vi "Self-Test.vi"(8 "error in (no error)":errorcluster, 11 "VISA resource name":refnum<visa-resource-name>) -> (0 "error out":errorcluster, 1 "Self-Test Result Message":string, 2 "Self-Test Result Code":i32, 3 "VISA resource name out":refnum<visa-resource-name>)   [LabVIEW 2014, in "Agilent U2000 Series.lvlib"]
doc: "Runs the instrument's self-test routine and returns the test results."
uses:
  Agilent U2000 Series.lvlib
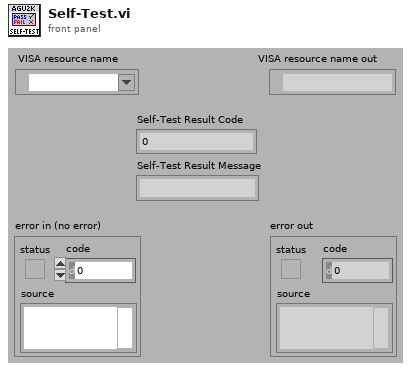
[diagram p1: front panel]
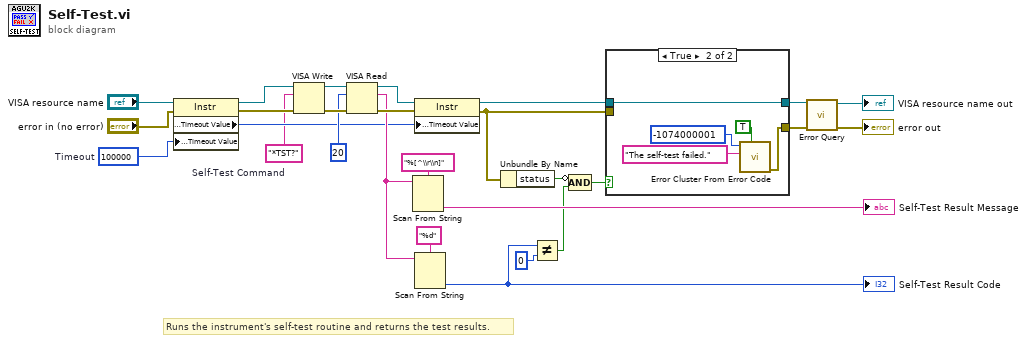
[diagram p0: block diagram]
diagram:
  w14 = u32 100000  # Timeout
  w10 = "*TST?"  # Self-Test Command
  # "Runs the instrument's self-test routine and returns the test results."
  n1 = property class="Instr"(reference="VISA resource name", error in="error in (no error)", "General Settings:Timeout Value"=w14) -> (reference out=w12:refnum<visa-resource-name>, error out=w13:errorcluster, "General Settings:Timeout Value"=w11:u32)
  n2 = VISA Write(VISA resource name=w12, write buffer=w10, error in (no error)=w13) -> (VISA resource name out=w23:refnum<visa-resource-name>, error out=w22:errorcluster)  [unwired: 1 out]
  n3 = VISA Read(VISA resource name=w23, byte count=u32 20 ("byte count (20)"), error in (no error)=w22) -> (VISA resource name out=w25:refnum<visa-resource-name>, read buffer=w18:string, error out=w24:errorcluster)  [unwired: 1 out]
  n4 = Scan From String(format string="%[^\\r\\n]" ("Format String"), input string=w18) -> (output 1=→"Self-Test Result Message":string)  [unwired: 2 in, 4 out]
  n5 = property class="Instr"(reference=w25, error in=w24, "General Settings:Timeout Value"=w11) -> (reference out=w9:refnum<visa-resource-name>, error out=w8:errorcluster)
  n6 = Scan From String(format string="%d", input string=w18) -> (output 1=w2:i32)  [unwired: 2 in, 4 out]
  "Self-Test Result Code" <- w2
  n7 = Unbundle By Name(w8) -> ("status"=w4:bool)
  n8 = Not Equal?(x=w2, y=0) -> (x != y?=w5:bool)
  n9 = Compound Arithmetic op=AND(invert w4, w5) -> (w3:bool)
  n10 = case shown="True" w3 {
    tunnel: w9 -> [w29 w34]
    tunnel: w8 -> [w28 _]
    tunnel: [w28 w30] -> w7
    tunnel: [w29 w34] -> w6
    frame False {
    }
    frame True {
      n11 = call "Error Cluster From Error Code.vi"("show call chain? (False)"=TRUE, "error message (\"\")"="The self-test failed." ("Source (VI Name)"), "error code (0)"=-1074000001 ("Code")) -> ("error out"=w30:errorcluster)  [unwired: 1 in, 5 out]
    }
  }
  n12 = call "Error Query.vi"("error in (no error)"=w7, "VISA resource name"=w6) -> ("error out"=→"error out":errorcluster, "VISA resource name out"=→"VISA resource name out":refnum<visa-resource-name>)  [unwired: 8 out]
